vi "linear_random_process.vi"(0 "A":T1, 1 "x0":T1, 5 "B":T1, 7 "C":T1, 11 "u":T1, 12 "v":T1, 13 "w":T1) -> (4 "y":T1, 15 "x":T1)   [LabVIEW 2016]
uses:
  <vilib>/Analysis/Matrix/Datatypes/RealMatrix.ctl
  <vilib>/Analysis/baseanly.llb/Real A x B.vi
  <vilib>/Analysis/Matrix/Numeric/Add/Add - RM,RM.vi
  <vilib>/Analysis/NI_AALBase.lvlib
  <vilib>/Analysis/Matrix/NI_Matrix.lvlib
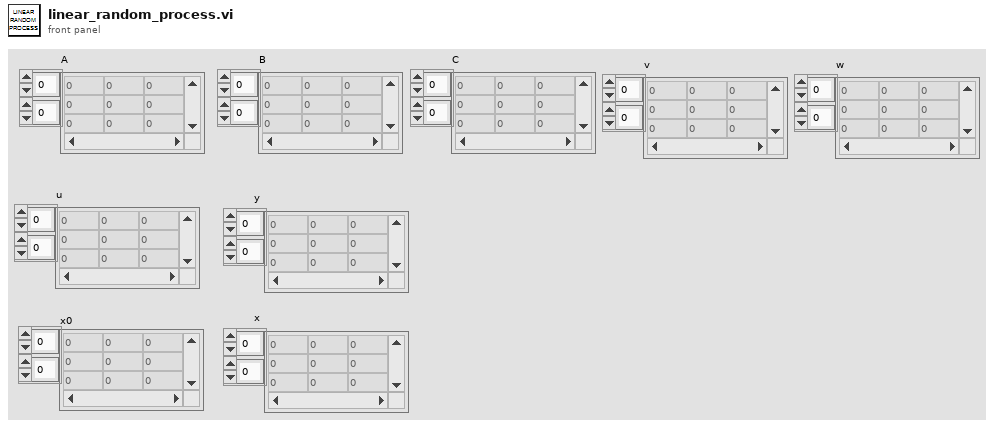
[diagram p1: front panel]
types:
  T1 = typedef "NI_Matrix.lvlib/RealMatrix.ctl" = dbl[][]
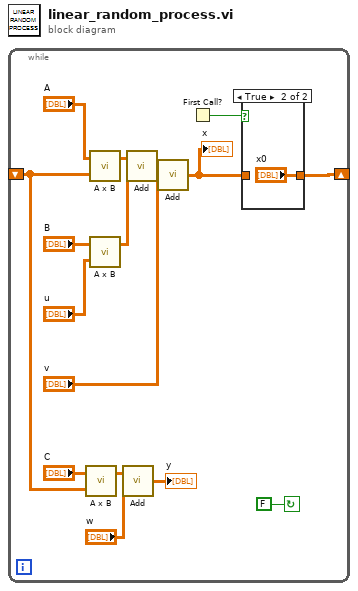
[diagram p0: block diagram]
diagram:
  n1 = while {
    shift-right: [w3] -> _
    shift-left: _ -> [w5]
    stop <- FALSE continue-if-true
    n2 = call-poly <vilib>:"A x B.vi"("B"=w5, "A"="C") -> ("A x B"=w7:T1)  [unwired: 1 out]
    n3 = call-poly <vilib>:"A x B.vi"("B"=w5, "A"="A") -> ("A x B"=w14:T1)  [unwired: 1 out]
    n4 = call-poly <vilib>:"A x B.vi"("B"="u", "A"="B") -> ("A x B"=w11:T1)  [unwired: 1 out]
    n5 = call-poly <vilib>:"Add.vi"("Real Matrix B"="w", "Real Matrix A"=w7) -> ("A + B"=→"y":T1)
    n6 = call-poly <vilib>:"Add.vi"("Real Matrix B"=w11, "Real Matrix A"=w14) -> ("A + B"=w10:T1)
    n7 = call-poly <vilib>:"Add.vi"("Real Matrix B"="v", "Real Matrix A"=w10) -> ("A + B"=w2:T1)
    "x" <- w2
    n8 = First Call?() -> (First Call?: T/F=w1:bool)
    n9 = case shown="True" w1 {
      tunnel: [w17 "x0"] -> w3
      tunnel: w2 -> [w17 _]
      frame False {
      }
      frame True {
      }
    }
  }
